vi "Set Row Values.vi"(7 "Sheet Name":string, 8 "error in":errorcluster, 9 "Values":variant[](array[variant]), 10 "Cell Address":string, 11 "SpreadsheetDoc":refnum<k24>) -> (0 "error out":errorcluster, 3 "SpreadsheetDoc out":refnum<k24>)   [LabVIEW 2019, in "Open Xml.lvlib"]
uses:
  Open Xml.lvlib
  D:/git/Open-Xml-LabVIEW/Source/DocumentFormat.OpenXml.dll
  DocumentFormat.OpenXml.dll
  d4d88da9-1970-4e76-91d6-38cee4cd592d.vi
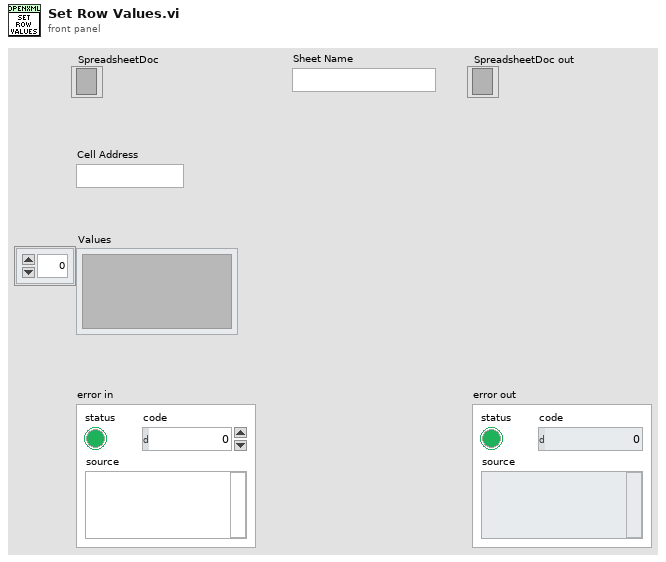
[diagram p1: front panel]
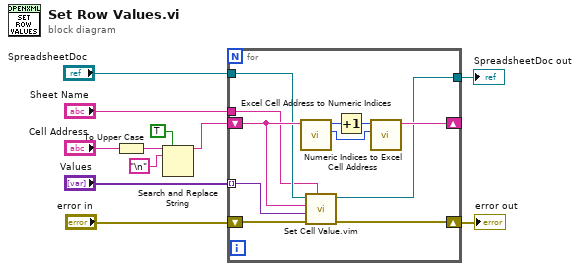
[diagram p0: block diagram]
diagram:
  n1 = To Upper Case(1:"Cell Address") -> (0:w4:string)
  n2 = Search and Replace String(replace all?=TRUE ("replace all? (F)"), input string=w4, search string="\n") -> (result string=w3:string)  [unwired: 5 in, 3 out]
  n3 = for {
    tunnel: "Values" -> [w18] mode=indexing
    shift-right: [w13] -> w11
    shift-left: "error in" -> [w17]
    shift-right: [w20] -> _
    shift-left: w3 -> [w16]
    tunnel: "SpreadsheetDoc" -> [w15]
    tunnel: [w14] -> w9
    tunnel: "Sheet Name" -> [w12]
    n4 = call "Excel Cell Address to Numeric Indices.vi"("Cell Name"=w16) -> ("Row Number"=w19:i32, "Column Number"=w22:i32)  [unwired: 9 in]
    n5 = call "Set Cell Value.vim"("Sheet Name"=w12, "error in"=w17, "Value"=w18, "Cell Address"=w16, "SpreadsheetDoc in"=w15) -> ("error out"=w13:errorcluster, "SpreadsheetDoc out"=w14:refnum<k24>)  [unwired: 5 in]
    n6 = Increment(x=w22) -> (x+1=w21:i32)
    n7 = call "Numeric Indices to Excel Cell Address.vi"("Row"=w19, "Column"=w21) -> ("Cell Address"=w20:string)  [unwired: 9 in]
  }
  "SpreadsheetDoc out" <- w9
  "error out" <- w11
